vi "Gaussian Window (CDB).vi"(10 "standard deviation":dbl=0.2, 11 "X":cdb[](array[numeric])) -> (0 "error":i32, 3 "Windowed X":cdb[](array[numeric]))   [LabVIEW 2017, in "NI_AALPro.lvlib"]
doc: "Applies an asymmetrical Gaussian window to the input sequence <B>X</B>. Wire data to the <B>X</B> input to determine the polymorphic instance to use or manually select the instance."
uses:
  <vilib>/Analysis/NI_AALPro.lvlib
  <resource>/lvanlys.dll
panel:
  # "Gaussian Window"
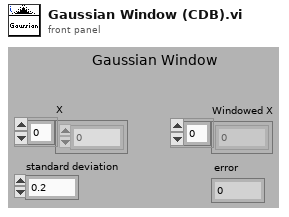
[diagram p1: front panel]
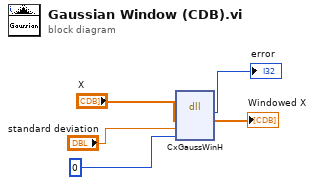
[diagram p0: block diagram]
diagram:
  n1 = dll-call lib="e:/builds/penguin/labview/branches/2017/dev/dist/resource/lvanlys.*" fn="CxGaussWinH"("X"="X", "stdDev"="standard deviation", "symmetric"=0) -> (→"error":i32, "X"=→"Windowed X":cdb[])  [unwired: 5 in, 2 out]
